vi "TDT-Wait For AI Buffer Space.vi"(0 "RPcox":refnum<k7>, 5 "Next Buffer":i32, 7 "Tag":string="ch2Index", 9 "Buffer Length":i32, 11 "error in (no error)":errorcluster, 12 "AI only":bool=TRUE) -> (4 "RPcox Out":refnum<k7>, 6 "Next Buffer Out":i32, 15 "error out":errorcluster)   [LabVIEW 2020]
uses:
  TDT-Globals.vi
panel:
  in  "Timeout (ms)":i32=5000
  out "Available":bool
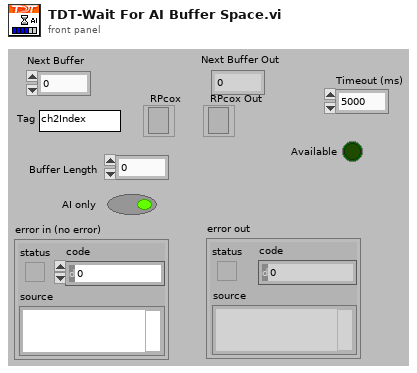
[diagram p1: front panel]
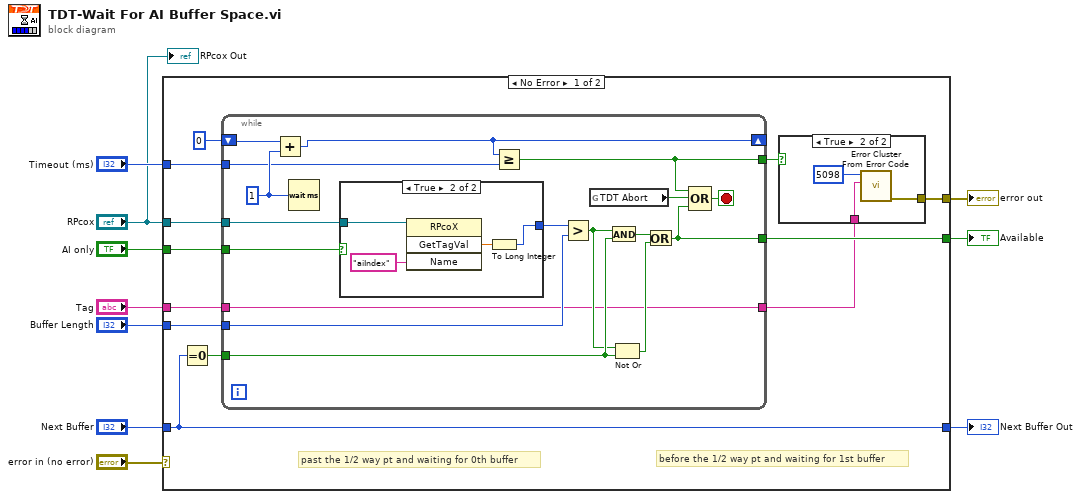
[diagram p0: block diagram]
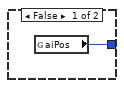
[diagram p3: hidden frame]
diagram:
  n1 = case shown="No Error" "error in (no error)" {
    selector: "error in (no error)" -> [_ w48]
    tunnel: [w13 w48] -> w9
    tunnel: "Buffer Length" -> [w22 _]
    tunnel: "Next Buffer" -> [w19 _]
    tunnel: [w20 _] -> w6
    tunnel: [w19 _] -> w5
    tunnel: "Tag" -> [w18 _]
    tunnel: "Timeout (ms)" -> [w16 _]
    tunnel: "RPcox" -> [w12 _]
    tunnel: "AI only" -> [w11 _]
    frame No Error {
      # "before the 1/2 way pt and waiting for 1st buffer"
      # "past the 1/2 way pt and waiting for 0th buffer"
      n2 = Equal To 0?(x=w19) -> (x = 0?=w21:bool)
      n3 = while {
        tunnel: w22 -> [w30]
        tunnel: w21 -> [w41]
        tunnel: [w37] -> w20
        tunnel: w18 -> [w29]
        shift-right: [w33] -> _
        shift-left: 0 -> [w35]
        tunnel: w16 -> [w32]
        tunnel: [w31] -> w15
        tunnel: [w29] -> w14
        tunnel: w12 -> [w28]
        tunnel: w11 -> [w26]
        stop <- w36 stop-if-true
        w34 = u32 1 ("milliseconds to wait")
        n4 = Add(x=w35, y=w34) -> (x+y=w33:u32)
        n5 = Wait (ms)(milliseconds to wait=w34) -> ()  [unwired: 1 out]
        n6 = case shown="True" w26 {
          tunnel: w28 -> [_ w47]
          tunnel: [w43 w44] -> w27
          frame False {
            n7 = global read "TDT-Globals.vi" "aiPos"() -> (w43:i32)
          }
          frame True {
            n8 = invoke class="RPcoX" method="GetTagVal"(reference=w47, "Name"="aiIndex" ("format string")) -> ("GetTagVal"=w45:sgl)  [unwired: 2 in, 3 out]
            n9 = To Long Integer(number=w45) -> (32bit integer=w44:i32)
          }
        }
        n10 = Greater Or Equal?(x=w33, y=w32) -> (x >= y?=w31:bool)
        n11 = Greater?(x=w27, y=w30) -> (0:w40:bool)
        n12 = global read "TDT-Globals.vi" "TDT Abort"() -> (w38:bool)
        n13 = And(x=w40, y=w41) -> (x .and. y?=w42:bool)
        n14 = Not Or(1:w41, 2:w40) -> (0:w39:bool)
        n15 = Or(x=w42, y=w39) -> (x .or. y?=w37:bool)
        n16 = Compound Arithmetic op=OR(w31, w38, w37) -> (w36:bool)
      }
      n17 = case shown="True" w15 {
        tunnel: w14 -> [_ w24]
        tunnel: [_ w23] -> w13
        frame False {
        }
        frame True {
          n18 = call <vilib>:"Error Cluster From Error Code.vi"("error message (\"\")"=w24, "error code (0)"=5098 ("specific error code to clear (0: all)")) -> ("error out"=w23:errorcluster)  [unwired: 7 in]
        }
      }
    }
    frame Error {
    }
  }
  "error out" <- w9
  "Next Buffer Out" <- w5
  "Available" <- w6
  "RPcox Out" <- "RPcox"
